vi "深大漂流记_main.vi"() -> ()   [LabVIEW 2018]
uses:
  <vilib>/Utility/file.llb/Read From Spreadsheet File (string).vi
panel:
  in  "富豪榜":i32[](listbox)
  out "leave":bool
  in  "关闭富豪榜":bool
  in  "查看富豪榜":bool
  in  "退出？":bool
  out "玩家":string caption="请输入你的大名"
  in  "放弃游戏":bool
  out "健康值":dbl(slide) scale=0.0..100.0
  out "当前健康值":i32=1000
  in  "医院":bool
  out "提示":string
  in  "信贷":bool
  out "欠债":i32
  in  "银行":bool
  out "存款":i32
  in  "演会中心":bool
  in  "机电学院":bool
  out "天数":i32
  out "余额":i32
  in  "饭堂":bool
  in  "图书馆":bool
  in  "库存":i32[](listbox)
  in  "卖出数量":i32 min=0 step=1
  in  "买入数量":i32 min=0 step=1
  in  "卖出":bool
  in  "买入":bool
  in  "商品价格":i32[](listbox)
  out "物品存在索引":i32[](array[numeric])
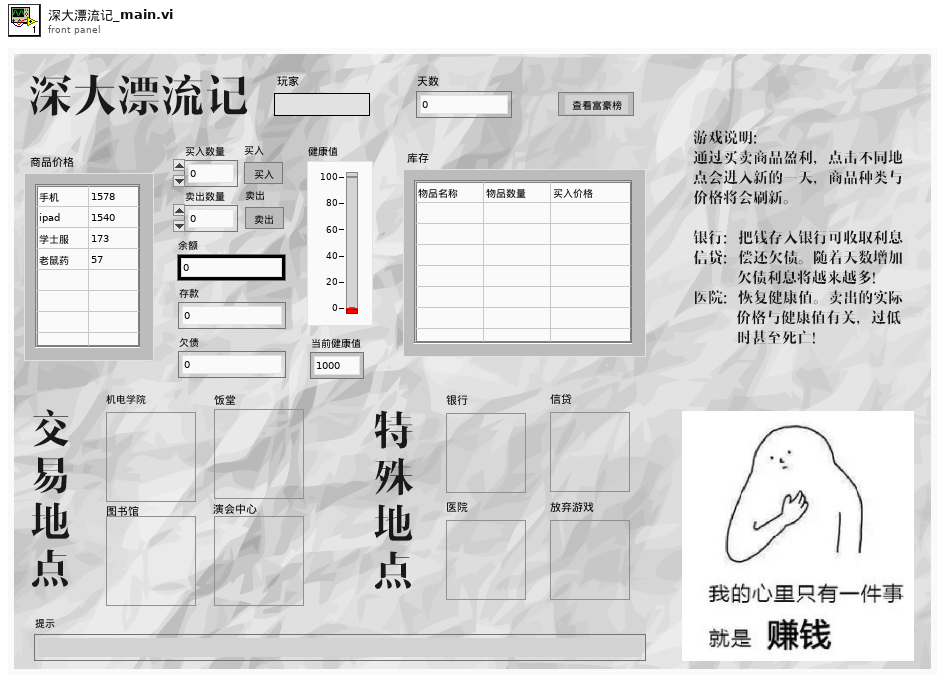
[diagram p1: front panel]
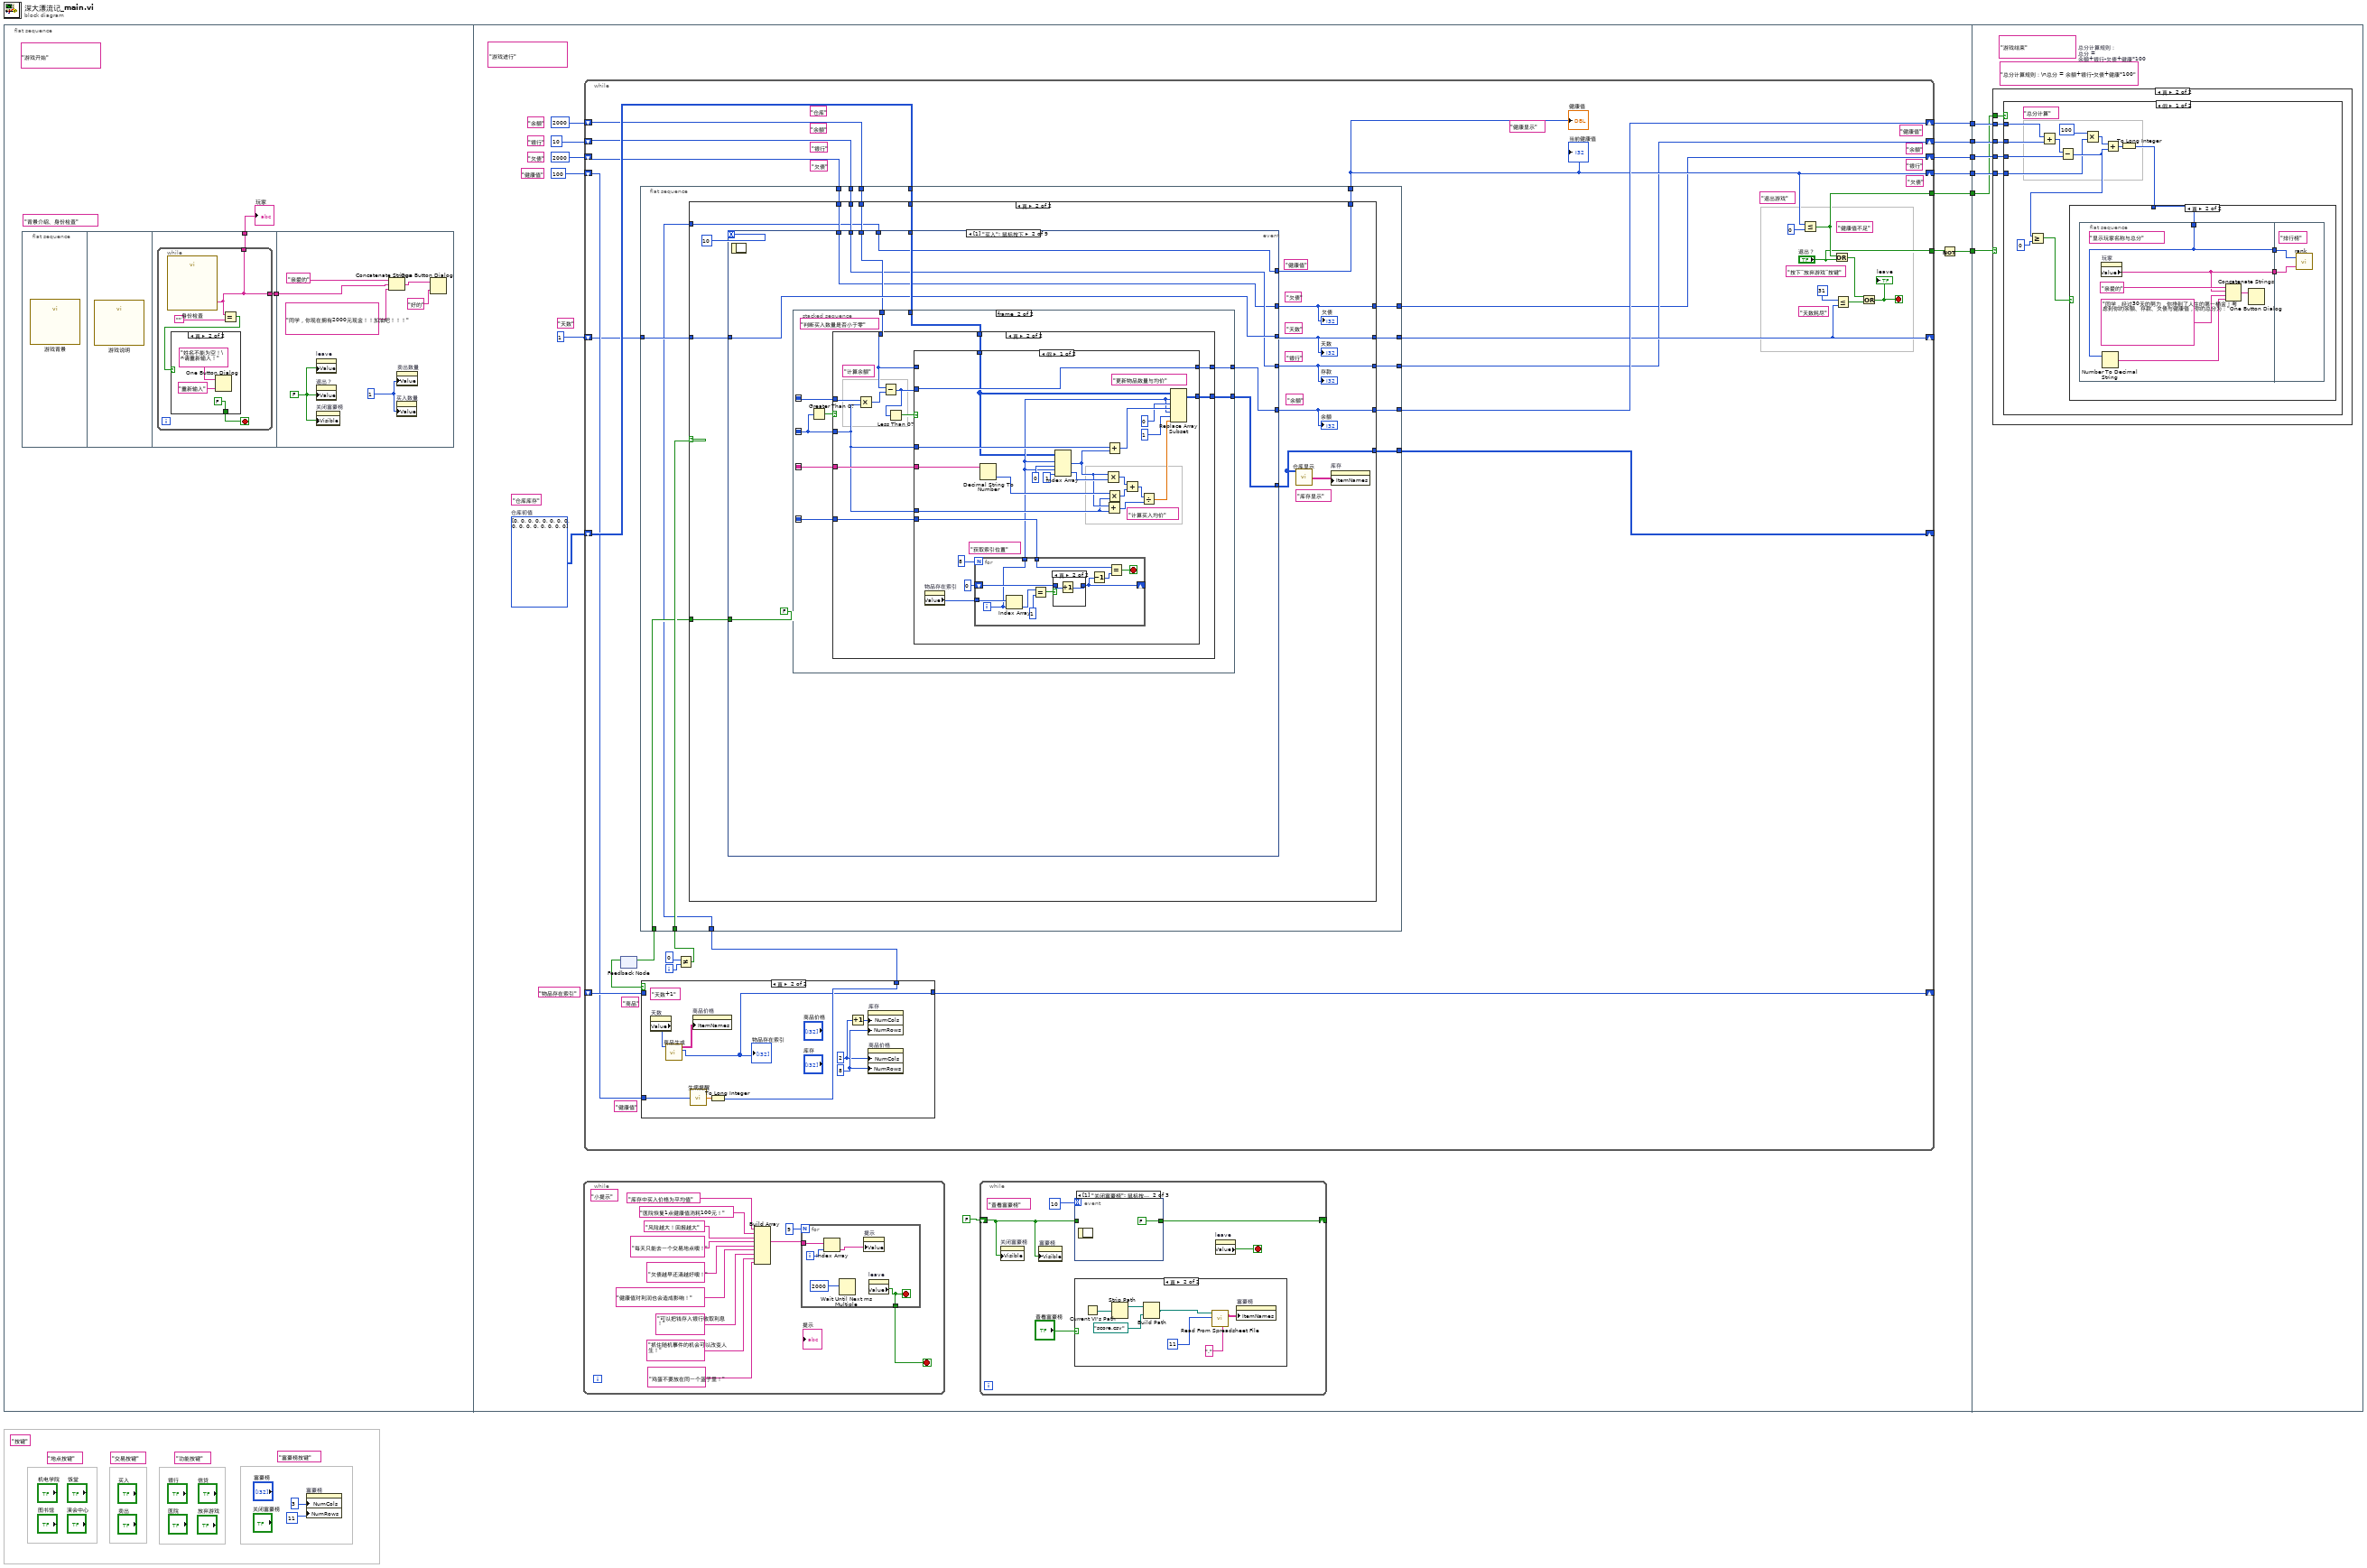
[diagram p0: block diagram]
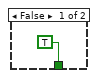
[diagram p2: hidden frame]
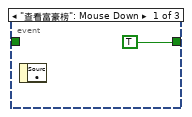
[diagram p3: hidden frame]
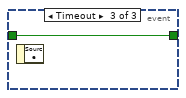
[diagram p4: hidden frame]
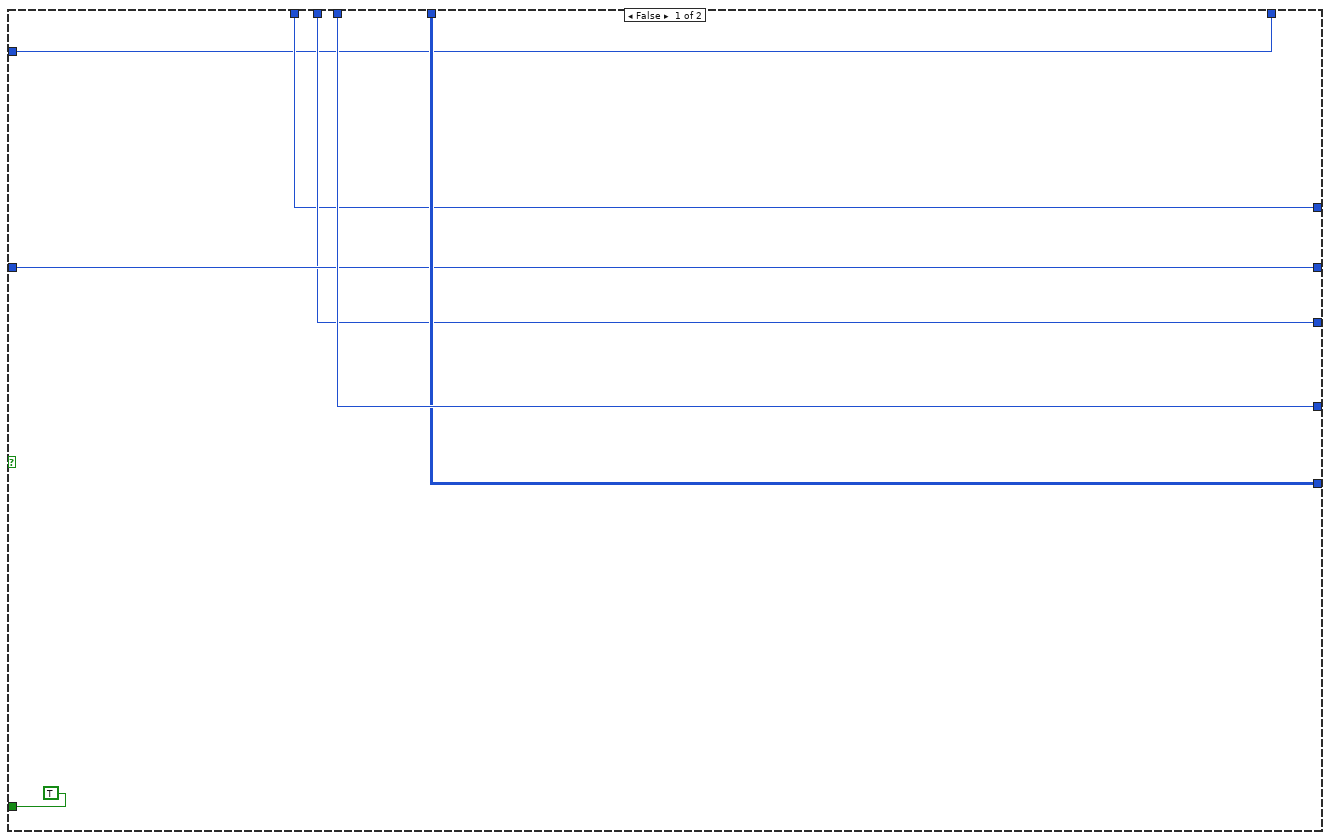
[diagram p7: hidden frame]
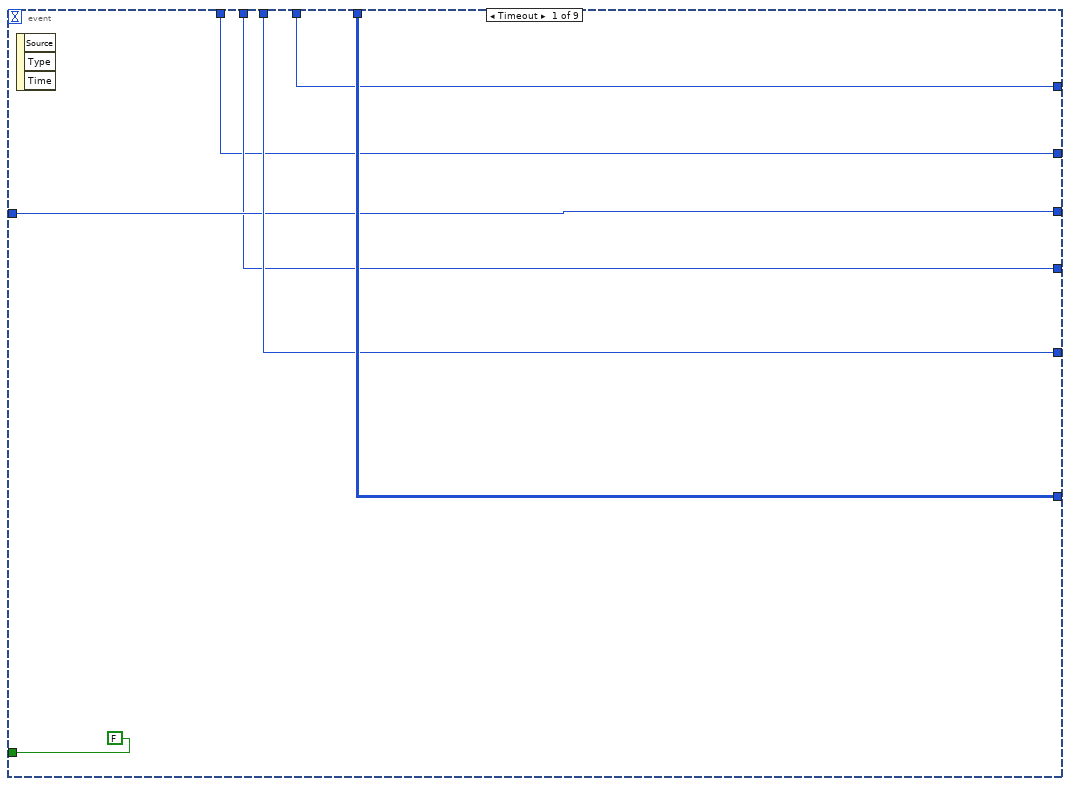
[diagram p8: hidden frame]
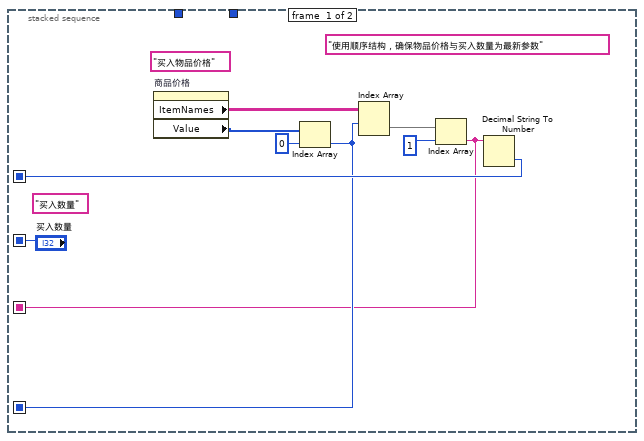
[diagram p9: hidden frame]
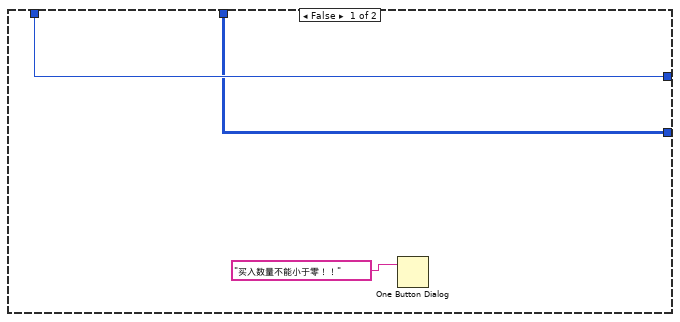
[diagram p10: hidden frame]
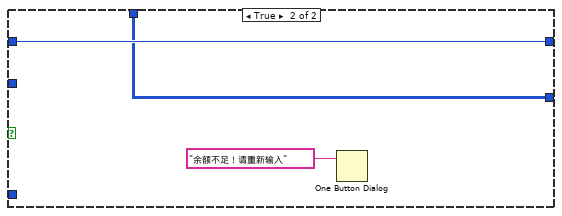
[diagram p12: hidden frame]
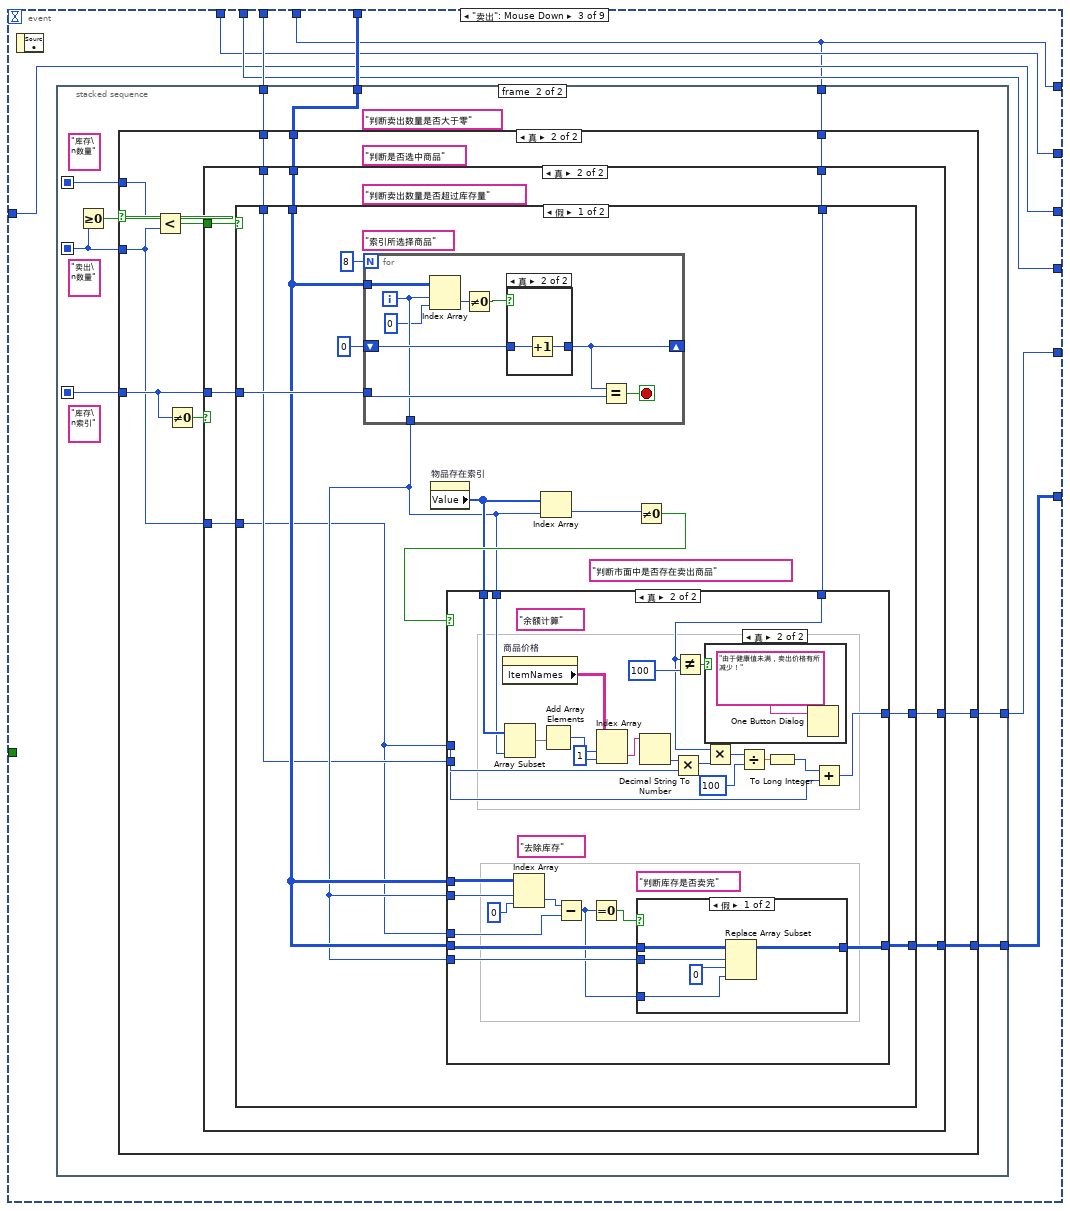
[diagram p13: hidden frame]
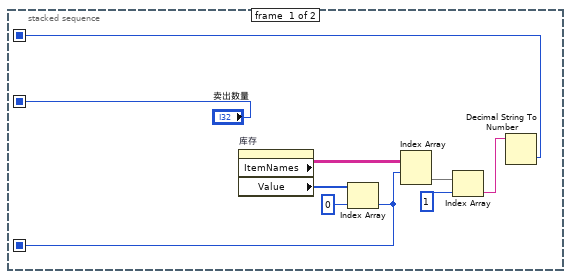
[diagram p14: hidden frame]
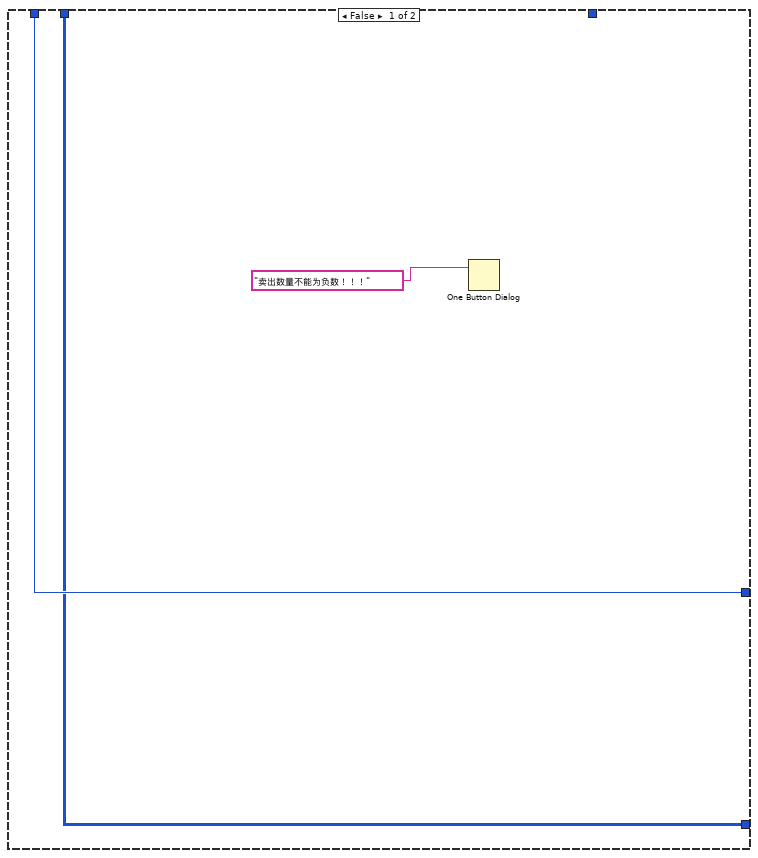
[diagram p15: hidden frame]
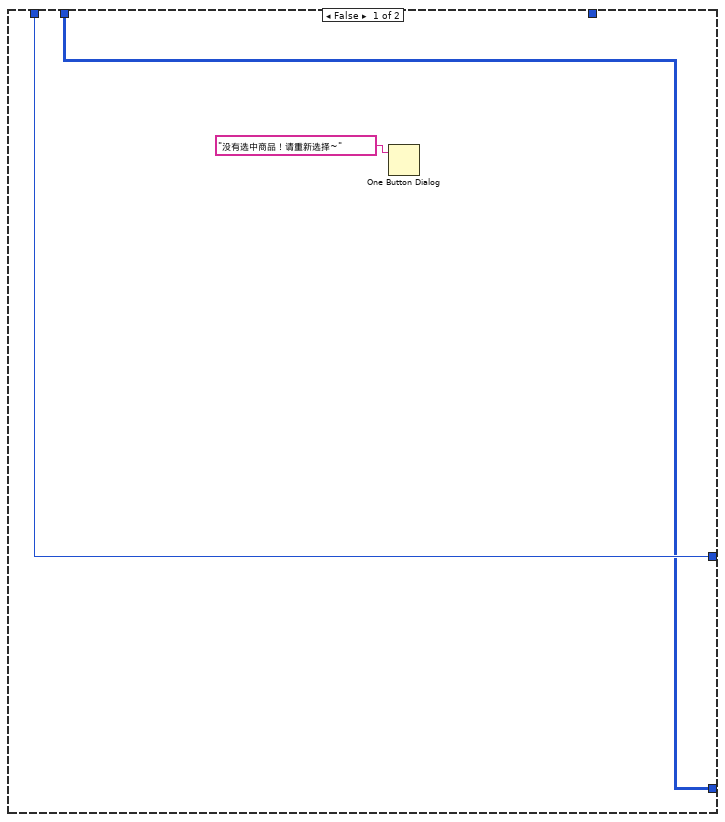
[diagram p16: hidden frame]
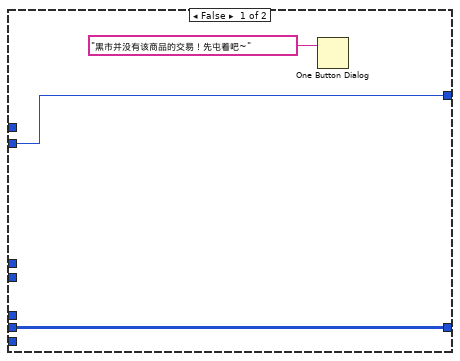
[diagram p17: hidden frame]
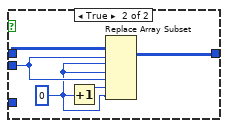
[diagram p19: hidden frame]
diagram:
  (unwired) "富豪榜按键"
  (unwired) "功能按键"
  (unwired) "交易按键"
  (unwired) "地点按键"
  (unwired) "按键"
  n1 = flat-sequence {
    tunnel: [w41] -> w8
    tunnel: [w40] -> w7
    tunnel: [w39] -> w6
    tunnel: [w38] -> w5
    tunnel: [w37] -> w4
    tunnel: [w28] -> w1
    tunnel: w8 -> [w522]
    tunnel: w7 -> [w521]
    tunnel: w6 -> [w520]
    tunnel: w5 -> [w519]
    tunnel: w4 -> [w518]
    tunnel: w1 -> [w517]
    frame #0 {
      (unwired) "背景介绍、身份检查"
      (unwired) "游戏开始"
      n2 = flat-sequence {
        tunnel: [w12] -> w10
        tunnel: [w11] -> w9
        tunnel: w10 -> [w26]
        frame #0 {
          n3 = call "游戏背景"() -> ()  [unwired: 18 in, 2 out]
        }
        frame #1 {
          n4 = call "游戏说明"() -> ()  [unwired: 18 in, 2 out]
        }
        frame #2 {
          n5 = while {
            tunnel: [w13] -> w12
            tunnel: [w13] -> w11
            stop <- w14 stop-if-true
            n6 = call "身份检查"() -> ("请输入你的姓名"=w13:string)  [unwired: 17 in, 2 out]
            n7 = Equal?(x=w13, y="") -> (x = y?=w15:bool)
            n8 = case shown="真" w15 {
              tunnel: [TRUE FALSE] -> w14
              frame False {
              }
              frame True {
                n9 = One Button Dialog(message="姓名不能为空！\n请重新输入！", button name ("OK")="重新输入" ("姓名输入提示")) -> ()  [unwired: 1 out]
              }
            }
          }
        }
        frame #3 {
          w21 = 1
          w22 = FALSE
          n10 = property on="leave" class="Bool (严格)"("Value"=w22) -> ()  [unwired: 2 in, 2 out]
          n11 = property on="退出？" class="Bool (严格)"("Value"=w22) -> ()  [unwired: 2 in, 2 out]
          n12 = property on="关闭富豪榜" class="Bool (严格)"("Visible"=w22) -> ()  [unwired: 2 in, 2 out]
          n13 = Concatenate Strings("亲爱的" ("姓名输入提示"), w26, "同学，你现在拥有2000元现金！！加油吧！！！" ("姓名输入提示")) -> (w24:string)
          n14 = property on="买入数量" class="DigNum (严格)"("Value"=w21) -> ()  [unwired: 2 in, 2 out]
          n15 = property on="卖出数量" class="DigNum (严格)"("Value"=w21) -> ()  [unwired: 2 in, 2 out]
          n16 = One Button Dialog(message=w24, button name ("OK")="好的" ("姓名输入提示")) -> ()  [unwired: 1 out]
        }
      }
      "玩家" <- w9
    }
    frame #1 {
      (unwired) "物品存在索引"
      (unwired) "游戏进行"
      (unwired) "健康值"
      (unwired) "欠债"
      (unwired) "银行"
      (unwired) "仓库库存"
      (unwired) "天数"
      (unwired) "余额"
      w32 = i32[][] [[0, 0], [0, 0], [0, 0], [0, 0], [0, 0], [0, 0], [0, 0], [0, 0]]  # 仓库初值
      n17 = while {
        stop <- w45 stop-if-true
        (unwired) "小提示"
        n18 = Build Array("库存中买入价格为平均值", "医院恢复1点健康值消耗100元！", "风险越大！回报越大", "每天只能去一个交易地点噢！", "欠债越早还清越好噢！", "健康值对利润也会造成影响！", "可以把钱存入银行收取利息！", "抓住随机事件的机会可以改变人生！", "鸡蛋不要放在同一个篮子里！") -> (w53:string[])
        n19 = for {
          N: 9 -> [_]
          tunnel: w53 -> [w58]
          tunnel: [w54] -> w45
          i -> [w57]
          stop <- w54 stop-if-true
          n20 = Index Array(array=w58, index=w57) -> (element=w55:string)
          n21 = Wait Until Next ms Multiple(millisecond multiple=2000) -> ()  [unwired: 1 out]
          n22 = property on="提示" class="Str"("Value"=w55) -> ()  [unwired: 2 in, 2 out]
          n23 = property on="leave" class="Bool (严格)"() -> ("Value"=w54:bool)  [unwired: 2 in, 2 out]
        }
      }
      n24 = while {
        shift-right: [w94] -> w41
        shift-left: 2000 -> [w87]
        shift-right: [w95] -> _
        shift-left: w32 -> [w96]
        shift-right: [w99] -> _
        shift-left: _ -> [w98]
        shift-right: [w91] -> _
        shift-left: 1 -> [w86]
        shift-right: [w79] -> w40
        shift-left: 10 -> [w88]
        shift-right: [w78] -> w39
        shift-left: 2000 -> [w89]
        shift-right: [w80] -> w38
        shift-left: 100 -> [w90]
        tunnel: [w81] -> w37
        tunnel: ["退出？"] -> w29
        i -> [w93]
        stop <- w84 stop-if-true
        (unwired) "天数耗尽"
        (unwired) "按下“放弃游戏”按键"
        (unwired) "健康值不足"
        (unwired) "退出游戏"
        (unwired) "健康显示"
        (unwired) "健康值"
        (unwired) "余额"
        (unwired) "银行"
        (unwired) "欠债"
        (unwired) "健康值"
        (unwired) "商品"
        (unwired) "仓库"
        (unwired) "余额"
        (unwired) "银行"
        (unwired) "欠债"
        n25 = feedback-in #1(w77) -> ()
        n26 = feedback #1() -> (w97:bool)  [unwired: 1 in]
        n27 = flat-sequence "平铺式顺序结构" {
          tunnel: w87 -> [w125]
          tunnel: [w121] -> w94
          tunnel: w76 -> [w124]
          tunnel: w96 -> [w123]
          tunnel: [w120] -> w95
          tunnel: [w122] -> w77
          tunnel: [w119] -> w91
          tunnel: w88 -> [w117]
          tunnel: [w116] -> w79
          tunnel: w89 -> [w115]
          tunnel: [w114] -> w78
          tunnel: [w113] -> w80
          tunnel: w75 -> [w112]
          tunnel: w86 -> [w118]
          frame #0 {
            n28 = case shown="真" w124 {
              tunnel: w125 -> [w132 w139]
              tunnel: [w132 w134] -> w121
              tunnel: w123 -> [w131 w146]
              tunnel: [w131 w144] -> w120
              tunnel: [TRUE w147] -> w122
              tunnel: [w129 w133] -> w119
              tunnel: w118 -> [w129 w142]
              tunnel: w117 -> [w128 w141]
              tunnel: [w128 w135] -> w116
              tunnel: w115 -> [w127 w140]
              tunnel: [w127 w136] -> w114
              tunnel: [w126 w138] -> w113
              tunnel: w112 -> [w126 w137]
              frame False {
              }
              frame True {
                (unwired) "库存显示"
                (unwired) "余额"
                (unwired) "天数"
                (unwired) "健康值"
                (unwired) "银行"
                (unwired) "欠债"
                n29 = event shown="[1] \"买入\": 鼠标按下" {
                  selector: _ -> [_ _ _ _ _ _ _ _ _]
                  dyn-events: _ -> [_ _ _ _ _ _ _ _ _]
                  timeout: 10 -> [_ _ _ _ _ _ _ _ _]
                  tunnel: [w152 w161 w242 w369 w378 w381 w447 w481 w512] -> w134
                  tunnel: w139 -> [w152 w158 w243 w369 w378 w386 w449 w482 w512]
                  tunnel: [w153 w162 w240 w370 w377 w382 w443 w486 w516] -> w144
                  tunnel: [FALSE FALSE _ TRUE FALSE _ _ _ _] -> w147
                  tunnel: w146 -> [w153 w163 w241 w370 w377 w382 w443 w486 w516]
                  tunnel: [w151 w159 w237 w365 w375 w380 w444 w483 w511] -> w133
                  tunnel: w142 -> [w151 w159 w237 w367 w375 w380 w444 w483 w511]
                  tunnel: w141 -> [w150 w157 w239 w357 w374 w385 w445 w484 w513]
                  tunnel: [w150 w157 w239 w358 w374 w384 w445 w484 w513] -> w135
                  tunnel: w140 -> [w149 w156 w238 w361 w373 w383 w448 w485 w514]
                  tunnel: [w149 w156 w238 w362 w373 w383 w446 w485 w514] -> w136
                  tunnel: w137 -> [w148 w155 w236 w366 w372 w379 w441 w478 w515]
                  tunnel: [w148 w155 w236 w366 w372 w379 w441 w477 w515] -> w138
                  event Timeout {
                    n30 = event-data() -> ()  [unwired: 1 in, 3 out]
                  }
                  event "买入": Mouse Down {
                    n31 = event-data() -> ()  [unwired: 1 in, 1 out]
                    n32 = stacked-sequence {
                      seq-local: ["买入数量" _] -> [_ w176]
                      seq-local: [w166 _] -> [_ w177]
                      seq-local: [w165 _] -> [_ w173]
                      seq-local: [w164 _] -> [_ w174]
                      tunnel: w158 -> [_ w181]
                      tunnel: w163 -> [_ w180]
                      tunnel: [_ w179] -> w162
                      tunnel: [_ w178] -> w161
                      frame #0 {
                        (unwired) "使用顺序结构，确保物品价格与买入数量为最新参数"
                        (unwired) "买入数量"
                        (unwired) "买入物品价格"
                        n33 = property on="商品价格" class="MCListbox (严格)"() -> ("ItemNames"=w169:string[][], "Value"=w168:i32[])  [unwired: 2 in, 2 out]
                        n34 = Index Array(array=w168, index=0) -> (element=w165:i32)
                        n35 = Index Array(array=w169, index (row)=w165) -> (element=w170:string[])  [unwired: 1 in]
                        n36 = Index Array(array=w170, index=1) -> (element=w164:string)
                        n37 = Decimal String To Number(string=w164) -> (number=w166:i32)  [unwired: 2 in, 1 out]
                      }
                      frame #1 {
                        (unwired) "判断买入数量是否小于零"
                        n38 = Greater Than 0?(x=w176) -> (x > 0?=w175:bool)
                        n39 = case shown="真" w175 {
                          tunnel: w181 -> [w183 w186]
                          tunnel: w174 -> [_ w194]
                          tunnel: w173 -> [_ w193]
                          tunnel: w180 -> [w182 w192]
                          tunnel: [w182 w191] -> w179
                          tunnel: [w183 w190] -> w178
                          tunnel: w177 -> [_ w189]
                          tunnel: w176 -> [_ w185]
                          frame False {
                            n40 = One Button Dialog(message="买入数量不能小于零！！") -> ()  [unwired: 1 in, 1 out]
                          }
                          frame True {
                            (unwired) "计算余额"
                            n41 = Multiply(x=w189, y=w185) -> (x*y=w195:i32)
                            n42 = Subtract(x=w186, y=w195) -> (x-y=w188:i32)
                            n43 = Less Than 0?(x=w188) -> (x < 0?=w187:bool)
                            n44 = case shown="假" w187 {
                              tunnel: [w219 w235] -> w190
                              tunnel: w188 -> [w219 _]
                              tunnel: w186 -> [_ w235]
                              tunnel: w194 -> [w213 _]
                              tunnel: w193 -> [w200 _]
                              tunnel: w192 -> [w196 w234]
                              tunnel: [w206 w234] -> w191
                              tunnel: w185 -> [w202 _]
                              tunnel: w185 -> [w199 _]
                              frame False {
                                (unwired) "更新物品数量与均价"
                                (unwired) "计算买入均价"
                                (unwired) "获取索引位置"
                                n45 = property on="物品存在索引" class="Arr (严格)"() -> ("Value"=w197:i32[])  [unwired: 2 in, 2 out]
                                n46 = for {
                                N: 8 -> [_]
                                tunnel: w197 -> [w229]
                                shift-right: [w225] -> _
                                shift-left: 0 -> [w226]
                                tunnel: w200 -> [w223]
                                tunnel: [w222] -> w198
                                i -> [w222]
                                stop <- w220 stop-if-true
                                n47 = Index Array(array=w229, index=w222) -> (element=w228:i32)
                                n48 = Equal?(x=w228, y=1) -> (x = y?=w221:bool)
                                n49 = case shown="真" w221 {
                                tunnel: w226 -> [w230 w232]
                                tunnel: [w230 w231] -> w225
                                frame False {
                                }
                                frame True {
                                n50 = Increment(x=w232) -> (x+1=w231:i32)
                                }
                                }
                                n51 = Decrement(x=w225) -> (x-1=w224:i32)
                                n52 = Equal?(x=w223, y=w224) -> (x = y?=w220:bool)
                                }
                                n53 = Decimal String To Number(string=w213) -> (number=w212:i32)  [unwired: 2 in, 1 out]
                                n54 = Index Array(array=w196, index (row) #1=w198, index (col) #1=0, index (row) #2=w198, index (col) #2=1) -> (element #1=w209:i32, element #2=w214:i32)
                                n55 = Multiply(x=w209, y=w214) -> (x*y=w211:i32)
                                n56 = Add(x=w209, y=w199) -> (x+y=w207:i32)
                                n57 = Add(x=w202, y=w209) -> (x+y=w216:i32)
                                n58 = Multiply(x=w212, y=w199) -> (x*y=w210:i32)
                                n59 = Add(x=w211, y=w210) -> (x+y=w208:i32)
                                n60 = Divide(x=w208, y=w207) -> (x/y=w203:dbl)
                                n61 = Replace Array Subset(array=w196, new element #1=w216, index (row) #1=w198, index (col) #1=0, new element #2=w203, index (row) #2=w198, index (col) #2=1) -> (w206:i32[][])
                              }
                              frame True {
                                n62 = One Button Dialog(message="余额不足！请重新输入") -> ()  [unwired: 1 in, 1 out]
                              }
                            }
                          }
                        }
                      }
                    }
                  }
                  event "卖出": Mouse Down {
                    n63 = event-data() -> ()  [unwired: 1 in, 1 out]
                    n64 = stacked-sequence {
                      seq-local: ["卖出数量" _] -> [_ w253]
                      seq-local: [w249 _] -> [_ w261]
                      seq-local: [w244 _] -> [_ w257]
                      tunnel: w241 -> [_ w260]
                      tunnel: w243 -> [_ w259]
                      tunnel: [_ w258] -> w242
                      tunnel: [_ w256] -> w240
                      tunnel: w236 -> [_ w255]
                      frame #0 {
                        n65 = property on="库存" class="MCListbox (严格)"() -> ("ItemNames"=w247:string[][], "Value"=w246:i32[])  [unwired: 2 in, 2 out]
                        n66 = Index Array(array=w246, index=0) -> (element=w244:i32)
                        n67 = Index Array(array=w247, index (row)=w244) -> (element=w248:string[])  [unwired: 1 in]
                        n68 = Index Array(array=w248, index=1) -> (element=w250:string)
                        n69 = Decimal String To Number(string=w250) -> (number=w249:i32)  [unwired: 2 in, 1 out]
                      }
                      frame #1 {
                        (unwired) "库存\n索引"
                        (unwired) "库存\n数量"
                        (unwired) "卖出\n数量"
                        (unwired) "判断卖出数量是否大于零"
                        n70 = Greater Or Equal To 0?(x=w253) -> (x >= 0?=w254:bool)
                        n71 = case shown="真" w254 {
                          tunnel: w261 -> [_ w274]
                          tunnel: w260 -> [w262 w272]
                          tunnel: w259 -> [w263 w271]
                          tunnel: [w263 w270] -> w258
                          tunnel: w257 -> [_ w269]
                          tunnel: w253 -> [_ w267]
                          tunnel: [w262 w266] -> w256
                          tunnel: w255 -> [_ w265]
                          frame False {
                            n72 = One Button Dialog(message="卖出数量不能为负数！！！") -> ()  [unwired: 1 in, 1 out]
                          }
                          frame True {
                            (unwired) "判断是否选中商品"
                            n73 = Less?(x=w274, y=w267) -> (x < y?=w273:bool)
                            n74 = Not Equal To 0?(x=w269) -> (x != 0?=w268:bool)
                            n75 = case shown="真" w268 {
                              tunnel: w273 -> [_ w281]
                              tunnel: w272 -> [w275 w285]
                              tunnel: w269 -> [_ w284]
                              tunnel: w267 -> [_ w283]
                              tunnel: w271 -> [w276 w278]
                              tunnel: [w276 w282] -> w270
                              tunnel: [w275 w280] -> w266
                              tunnel: w265 -> [_ w279]
                              frame False {
                                n76 = One Button Dialog(message="没有选中商品！请重新选择~") -> ()  [unwired: 1 in, 1 out]
                              }
                              frame True {
                                (unwired) "判断卖出数量是否超过库存量"
                                n77 = case shown="假" w281 {
                                tunnel: w285 -> [w291 w355]
                                tunnel: w284 -> [w296 _]
                                tunnel: w283 -> [w286 _]
                                tunnel: [w292 w354] -> w282
                                tunnel: [w289 w355] -> w280
                                tunnel: w279 -> [w288 _]
                                tunnel: w278 -> [w287 w354]
                                frame False {
                                (unwired) "判断市面中是否存在卖出商品"
                                (unwired) "索引所选择商品"
                                n78 = for {
                                N: 8 -> [_]
                                tunnel: w291 -> [w346]
                                shift-right: [w348] -> _
                                shift-left: 0 -> [w344]
                                tunnel: w296 -> [w345]
                                tunnel: [w343] -> w290
                                i -> [w343]
                                stop <- w347 stop-if-true
                                n79 = Index Array(array=w346, index (row)=w343, index (col)=0) -> (element=w350:i32)
                                n80 = Not Equal To 0?(x=w350) -> (x != 0?=w349:bool)
                                n81 = case shown="真" w349 {
                                tunnel: [w351 w353] -> w348
                                tunnel: w344 -> [w351 w352]
                                frame False {
                                }
                                frame True {
                                n82 = Increment(x=w352) -> (x+1=w353:i32)
                                }
                                }
                                n83 = Equal?(x=w348, y=w345) -> (x = y?=w347:bool)
                                }
                                n84 = property on="物品存在索引" class="Arr (严格)"() -> ("Value"=w293:i32[])  [unwired: 2 in, 2 out]
                                n85 = Index Array(array=w293, index=w290) -> (element=w295:i32)
                                n86 = Not Equal To 0?(x=w295) -> (x != 0?=w294:bool)
                                n87 = case shown="真" w294 {
                                tunnel: w290 -> [_ w329]
                                tunnel: w293 -> [_ w330]
                                tunnel: w286 -> [_ w324]
                                tunnel: w287 -> [w300 w323]
                                tunnel: [w300 w322] -> w292
                                tunnel: w291 -> [_ w320]
                                tunnel: w290 -> [_ w319]
                                tunnel: w286 -> [_ w317]
                                tunnel: w291 -> [w299 w314]
                                tunnel: w290 -> [_ w313]
                                tunnel: [w299 w312] -> w289
                                tunnel: w288 -> [_ w302]
                                frame False {
                                n88 = One Button Dialog(message="黑市并没有该商品的交易！先屯着吧~") -> ()  [unwired: 1 in, 1 out]
                                }
                                frame True {
                                (unwired) "判断库存是否卖完"
                                (unwired) "去除库存"
                                (unwired) "余额计算"
                                n89 = property on="商品价格" class="MCListbox (严格)"() -> ("ItemNames"=w327:string[][])  [unwired: 2 in, 2 out]
                                n90 = Array Subset(array=w330, length=w329) -> (w328:i32[])  [unwired: 1 in]
                                n91 = Index Array(array=w320, index (row)=w319, index (col)=0) -> (element=w316:i32)
                                n92 = Add Array Elements(numeric array=w328) -> (sum=w326:i32)
                                n93 = Subtract(x=w316, y=w317) -> (x-y=w311:i32)
                                n94 = Equal To 0?(x=w311) -> (x = 0?=w315:bool)
                                n95 = Index Array(array=w327, index (row)=w326, index (col)=1) -> (element=w307:string)
                                n96 = case shown="假" w315 {
                                tunnel: w314 -> [w336 w341]
                                tunnel: w313 -> [w335 w340]
                                tunnel: [w332 w337] -> w312
                                tunnel: w311 -> [w333 _]
                                frame False {
                                n97 = Replace Array Subset(array=w336, new element=w333, index (row)=w335, index (col)=0) -> (w332:i32[][])
                                }
                                frame True {
                                w338 = 0
                                n98 = Increment(x=w338) -> (x+1=w339:i32)
                                n99 = Replace Array Subset(array=w341, new element #1=w338, index (row) #1=w340, index (col) #1=w338, new element #2=w338, index (row) #2=w340, index (col) #2=w339) -> (w337:i32[][])
                                }
                                }
                                n100 = Decimal String To Number(string=w307) -> (number=w321:i32)  [unwired: 2 in, 1 out]
                                n101 = Multiply(x=w321, y=w324) -> (x*y=w310:i32)
                                n102 = Not Equal?(x=w302, y=100) -> (x != y?=w304:bool)
                                n103 = case shown="真" w304 {
                                frame False {
                                }
                                frame True {
                                n104 = One Button Dialog(message="由于健康值未满，卖出价格有所减少！") -> ()  [unwired: 1 in, 1 out]
                                }
                                }
                                n105 = Multiply(x=w302, y=w310) -> (x*y=w308:i32)
                                n106 = Divide(x=w308, y=100) -> (x/y=w306:dbl)
                                n107 = To Long Integer(number=w306) -> (32bit integer=w305:i32)
                                n108 = Add(x=w305, y=w323) -> (x+y=w322:i32)
                                }
                                }
                                }
                                frame True {
                                n109 = One Button Dialog(message="库存太少啦！请重新选择~") -> ()  [unwired: 1 in, 1 out]
                                }
                                }
                              }
                            }
                          }
                        }
                      }
                    }
                  }
                  event "图书馆", "机电学院", "演会中心", "饭堂": Mouse Up {
                    n110 = event-data() -> ()  [unwired: 1 in, 8 out]
                    n111 = Add(x=1, y=w367) -> (x+y=w365:i32)
                    n112 = Multiply(x=w357, y=1.05) -> (x*y=w359:dbl)
                    n113 = Multiply(x=w361, y=1.1) -> (x*y=w363:dbl)
                    n114 = To Long Integer(number=w359) -> (32bit integer=w358:i32)
                    n115 = To Long Integer(number=w363) -> (32bit integer=w362:i32)
                  }
                  event "库存", "商品价格": Mouse Down {
                    n116 = event-data() -> ()  [unwired: 1 in, 8 out]
                  }
                  event "银行": Mouse Down {
                    n117 = event-data() -> ()  [unwired: 1 in, 1 out]
                    n118 = Two Button Dialog(message="欢迎来到 IronBank ，你打算干什么？", 1:"取款", 2:"存款") -> (T button?=w387:bool)
                    n119 = case shown="假" w387 {
                      tunnel: w386 -> [w397 w421]
                      tunnel: w385 -> [w396 w420]
                      tunnel: [w395 w419] -> w381
                      tunnel: [w394 w418] -> w384
                      frame False {
                        (unwired) "取款"
                        n120 = call "输入取款数额"() -> ("取款数额"=w392:dbl)  [unwired: 17 in, 2 out]
                        n121 = To Long Integer(number=w392) -> (32bit integer=w391:i32)
                        n122 = Greater Or Equal To 0?(x=w391) -> (x >= 0?=w393:bool)
                        n123 = case shown="真" w393 {
                          tunnel: w397 -> [w400 w405]
                          tunnel: w396 -> [w399 w402]
                          tunnel: [w399 w404] -> w395
                          tunnel: [w400 w403] -> w394
                          tunnel: w391 -> [_ w401]
                          frame False {
                            n124 = One Button Dialog(message="取款数额必须大于等于0！") -> ()  [unwired: 1 in, 1 out]
                          }
                          frame True {
                            n125 = Less?(x=w402, y=w401) -> (x < y?=w406:bool)
                            n126 = case shown="假" w406 {
                              tunnel: [w411 w412] -> w404
                              tunnel: [w410 w413] -> w403
                              tunnel: w401 -> [w409 _]
                              tunnel: w405 -> [w408 w412]
                              tunnel: w402 -> [w407 w413]
                              frame False {
                                n127 = Subtract(x=w407, y=w409) -> (x-y=w410:i32)
                                n128 = Add(x=w408, y=w409) -> (x+y=w411:i32)
                              }
                              frame True {
                                n129 = One Button Dialog(message="余额不足！请重新输入") -> ()  [unwired: 1 in, 1 out]
                              }
                            }
                          }
                        }
                      }
                      frame True {
                        (unwired) "存款"
                        n130 = call "输入存款数额"() -> ("存款数额"=w416:dbl)  [unwired: 17 in, 2 out]
                        n131 = To Long Integer(number=w416) -> (32bit integer=w415:i32)
                        n132 = Greater Or Equal To 0?(x=w415) -> (x >= 0?=w417:bool)
                        n133 = case shown="真" w417 {
                          tunnel: w421 -> [w422 w429]
                          tunnel: w420 -> [w423 w428]
                          tunnel: [w422 w427] -> w419
                          tunnel: [w423 w426] -> w418
                          tunnel: w415 -> [_ w425]
                          frame False {
                            n134 = One Button Dialog(message="存款数额必须大于等于0！") -> ()  [unwired: 1 in, 1 out]
                          }
                          frame True {
                            n135 = Less?(x=w429, y=w425) -> (x < y?=w430:bool)
                            n136 = case shown="假" w430 {
                              tunnel: w425 -> [w435 _]
                              tunnel: [w434 w437] -> w427
                              tunnel: [w433 w436] -> w426
                              tunnel: w429 -> [w432 w437]
                              tunnel: w428 -> [w431 w436]
                              frame False {
                                n137 = Add(x=w431, y=w435) -> (x+y=w433:i32)
                                n138 = Subtract(x=w432, y=w435) -> (x-y=w434:i32)
                              }
                              frame True {
                                n139 = One Button Dialog(message="余额不足！请重新输入") -> ()  [unwired: 1 in, 1 out]
                              }
                            }
                          }
                        }
                      }
                    }
                  }
                  event "信贷": Mouse Down {
                    n140 = event-data() -> ()  [unwired: 1 in, 1 out]
                    n141 = call "输入还钱数额"() -> ("还钱数额"=w440:dbl)  [unwired: 17 in, 2 out]
                    n142 = To Long Integer(number=w440) -> (32bit integer=w439:i32)
                    n143 = Greater Or Equal To 0?(x=w439) -> (x >= 0?=w442:bool)
                    n144 = case shown="真" w442 {
                      tunnel: w449 -> [w451 w457]
                      tunnel: w439 -> [_ w456]
                      tunnel: w448 -> [w452 w455]
                      tunnel: [w451 w454] -> w447
                      tunnel: [w452 w453] -> w446
                      frame False {
                        n145 = One Button Dialog(message="输入必须大于等于0！") -> ()  [unwired: 1 in, 1 out]
                      }
                      frame True {
                        n146 = Less?(x=w457, y=w456) -> (x < y?=w458:bool)
                        n147 = case shown="假" w458 {
                          tunnel: w457 -> [w463 w475]
                          tunnel: w456 -> [w459 _]
                          tunnel: w455 -> [w462 w474]
                          tunnel: [w461 w475] -> w454
                          tunnel: [w460 w474] -> w453
                          frame False {
                            n148 = Less?(x=w462, y=w459) -> (x < y?=w464:bool)
                            n149 = case shown="假" w464 {
                              tunnel: w463 -> [w469 w473]
                              tunnel: w462 -> [w468 w472]
                              tunnel: [w466 w471] -> w461
                              tunnel: [w465 0] -> w460
                              tunnel: w459 -> [w467 _]
                              frame False {
                                n150 = Subtract(x=w469, y=w467) -> (x-y=w466:i32)
                                n151 = Subtract(x=w468, y=w467) -> (x-y=w465:i32)
                              }
                              frame True {
                                n152 = Subtract(x=w473, y=w472) -> (x-y=w471:i32)
                              }
                            }
                          }
                          frame True {
                            n153 = One Button Dialog(message="余额不足！请重新输入！") -> ()  [unwired: 1 in, 1 out]
                          }
                        }
                      }
                    }
                  }
                  event "医院": Mouse Down {
                    w479 = 100  # 健康初值
                    n154 = event-data() -> ()  [unwired: 1 in, 1 out]
                    n155 = Not Equal?(x=w479, y=w478) -> (x != y?=w480:bool)
                    n156 = case shown="真" w480 {
                      tunnel: w482 -> [w489 w494]
                      tunnel: [w489 w490] -> w481
                      tunnel: w478 -> [w487 w492]
                      tunnel: [w487 w491] -> w477
                      frame False {
                        n157 = One Button Dialog(message="没病来什么医院！" ("姓名输入提示")) -> ()  [unwired: 1 in, 1 out]
                      }
                      frame True {
                        w496 = 100  # 医院花费倍数
                        w498 = 100  # 健康初值
                        n158 = Subtract(x=w498, y=w492) -> (x-y=w497:i32)
                        n159 = Multiply(x=w497, y=w496) -> (x*y=w495:i32)
                        n160 = Greater Or Equal?(x=w494, y=w495) -> (x >= y?=w493:bool)
                        n161 = case shown="真" w493 {
                          tunnel: w494 -> [w500 w509]
                          tunnel: [w500 w508] -> w490
                          tunnel: w495 -> [_ w503]
                          tunnel: w492 -> [w499 _]
                          tunnel: [w499 100] -> w491
                          frame False {
                            n162 = One Button Dialog(message="没钱看什么病！" ("姓名输入提示")) -> ()  [unwired: 1 in, 1 out]
                          }
                          frame True {
                            n163 = Number To Decimal String(number=w503) -> (decimal integer string=w504:string)  [unwired: 1 in]
                            n164 = Subtract(x=w509, y=w503) -> (x-y=w508:i32)
                            n165 = Concatenate Strings("医生开了点药给您，共花费了" ("姓名输入提示"), w504, "元！" ("姓名输入提示")) -> (w507:string)
                            n166 = One Button Dialog(message=w507) -> ()  [unwired: 1 in, 1 out]
                          }
                        }
                      }
                    }
                  }
                  event "放弃游戏": Mouse Down {
                    n167 = event-data() -> ()  [unwired: 1 in, 1 out]
                    n168 = property on="退出？" class="Bool (严格)"("Value"=TRUE) -> ()  [unwired: 2 in, 2 out]
                  }
                }
                "余额" <- w134
                "天数" <- w133
                "存款" <- w135
                "欠债" <- w136
                n169 = call "仓库显示.vi"("仓库"=w144) -> ("显示栏"=w143:string[][])  [unwired: 10 in]
                n170 = property on="库存" class="MCListbox (严格)"("ItemNames"=w143) -> ()  [unwired: 2 in, 2 out]
              }
            }
          }
        }
        n171 = case shown="真" w97 {
          tunnel: [w102 w104] -> w99
          tunnel: w98 -> [w102 _]
          tunnel: w90 -> [w101 w108]
          tunnel: [w101 w106] -> w75
          frame False {
          }
          frame True {
            (unwired) "天数+1"
            w111 = i8 8
            w109 = i8 2
            n172 = property on="天数" class="DigNum (严格)"() -> ("Value"=w103:i32)  [unwired: 2 in, 2 out]
            n173 = call "商品生成.vi"("天数"=w103) -> ("物品存在索引"=w104:i32[], "市面商品"=w105:string[][])  [unwired: 9 in]
            "物品存在索引" <- w104
            n174 = call "生病提醒.vi"("数值"=w108) -> ("数值 2"=w107:dbl)
            n175 = property on="商品价格" class="MCListbox (严格)"("ItemNames"=w105) -> ()  [unwired: 2 in, 2 out]
            n176 = To Long Integer(number=w107) -> (32bit integer=w106:i32)
            n177 = Increment(x=w109) -> (x+1=w110:i8)
            n178 = property on="库存" class="MCListbox (严格)"("NumCols"=w110, "NumRows"=w111) -> ()  [unwired: 2 in, 2 out]
            n179 = property on="商品价格" class="MCListbox (严格)"("NumCols"=w109, "NumRows"=w111) -> ()  [unwired: 2 in, 2 out]
          }
        }
        n180 = Not Equal?(x=0, y=w93) -> (x != y?=w76:bool)
        n181 = Less Or Equal?(x=w80, y=0) -> (x <= y?=w81:bool)
        n182 = Or(x=w81, y="退出？") -> (x .or. y?=w82:bool)
        n183 = Less Or Equal?(x=31, y=w91) -> (x <= y?=w85:bool)
        n184 = Or(x=w82, y=w85) -> (x .or. y?=w84:bool)
        "leave" <- w84
        "当前健康值" <- w80
        "健康值" <- w80
      }
      n185 = while {
        shift-right: [w60] -> _
        shift-left: FALSE -> [w59]
        stop <- w61 stop-if-true
        (unwired) "查看富豪榜"
        n186 = property on="关闭富豪榜" class="Bool (严格)"("Visible"=w59) -> ()  [unwired: 2 in, 2 out]
        n187 = property on="富豪榜" class="MCListbox (严格)"("Visible"=w59) -> ()  [unwired: 2 in, 2 out]
        n188 = event shown="[1] \"关闭富豪榜\": 鼠标按下" {
          selector: _ -> [_ _ _]
          dyn-events: _ -> [_ _ _]
          timeout: 10 -> [_ _ _]
          tunnel: w59 -> [_ _ w66]
          tunnel: [TRUE FALSE w66] -> w60
          event "查看富豪榜": Mouse Down {
            n189 = event-data() -> ()  [unwired: 1 in, 1 out]
          }
          event "关闭富豪榜": Mouse Down {
            n190 = event-data() -> ()  [unwired: 1 in, 1 out]
          }
          event Timeout {
            n191 = event-data() -> ()  [unwired: 1 in, 1 out]
          }
        }
        n192 = case shown="真" "查看富豪榜" {
          frame False {
          }
          frame True {
            n193 = Current VI's Path() -> (path=w71:path)
            n194 = Strip Path(path=w71) -> (stripped path=w70:path)  [unwired: 1 out]
            n195 = Build Path(base path=w70, name or relative path=path "score.csv") -> (appended path=w68:path)
            n196 = call-poly <vilib>:"Read From Spreadsheet File.vi"("delimiter (\\t)"=",", "number of rows (all:-1)"=11, "file path (dialog if empty)"=w68) -> ("all rows"=w67:string[][])  [unwired: 4 in, 4 out]
            n197 = property on="富豪榜" class="MCListbox (严格)"("ItemNames"=w67) -> ()  [unwired: 2 in, 2 out]
          }
        }
        n198 = property on="leave" class="Bool (严格)"() -> ("Value"=w61:bool)  [unwired: 2 in, 2 out]
      }
      n199 = Not(x=w29) -> (.not. x?=w28:bool)
    }
    frame #2 {
      (unwired) "总分计算规则：\n总分 = 余额+银行-欠债+健康*100"  # 总分计算规则： 总分 = 余额+银行-欠债+健康*100
      (unwired) "游戏结束"
      n200 = case shown="真" w517 {
        tunnel: w522 -> [_ w531]
        tunnel: w521 -> [_ w530]
        tunnel: w520 -> [_ w529]
        tunnel: w519 -> [_ w528]
        tunnel: w518 -> [_ w527]
        frame False {
          n201 = property on="玩家" class="Str"() -> ("Value"=w523:string)  [unwired: 2 in, 2 out]
          n202 = Concatenate Strings("亲爱的", w523, "同学，你点击了放弃游戏！重新开始请点击”运行“按钮！") -> (w524:string)
          n203 = One Button Dialog(message=w524) -> ()  [unwired: 1 in, 1 out]
        }
        frame True {
          n204 = case shown="假" w527 {
            tunnel: w531 -> [w542 _]
            tunnel: w530 -> [w541 _]
            tunnel: w529 -> [w540 _]
            tunnel: w528 -> [w532 _]
            frame False {
              (unwired) "总分计算"
              n205 = Add(x=w542, y=w541) -> (x+y=w543:i32)
              n206 = Subtract(x=w543, y=w540) -> (x-y=w533:i32)
              n207 = Greater Or Equal?(x=w533, y=0) -> (x >= y?=w534:bool)
              n208 = Multiply(x=100, y=w532) -> (x*y=w537:i32)
              n209 = Add(x=w537, y=w533) -> (x+y=w539:i32)
              n210 = To Long Integer(number=w539) -> (32bit integer=w536:i32)
              n211 = case shown="真" w534 {
                tunnel: w536 -> [_ w548]
                frame False {
                  n212 = property on="玩家" class="Str"() -> ("Value"=w544:string)  [unwired: 2 in, 2 out]
                  n213 = Concatenate Strings("亲爱的", w544, "同学，你破产了！游戏结束！") -> (w545:string)
                  n214 = One Button Dialog(message=w545) -> ()  [unwired: 1 in, 1 out]
                }
                frame True {
                  n215 = flat-sequence {
                    tunnel: w548 -> [w551]
                    tunnel: [w552] -> w550
                    tunnel: [w551] -> w549
                    tunnel: w550 -> [w558]
                    tunnel: w549 -> [w557]
                    frame #0 {
                      (unwired) "显示玩家名称与总分"
                      n216 = property on="玩家" class="Str"() -> ("Value"=w552:string)  [unwired: 2 in, 2 out]
                      n217 = Number To Decimal String(number=w551) -> (decimal integer string=w554:string)  [unwired: 1 in]
                      n218 = Concatenate Strings("亲爱的", w552, "同学，经过30天的努力，你挣到了人生的第一桶金！考虑到你的余额、存款、欠债与健康值，你的总分为：", w554) -> (w553:string)
                      n219 = One Button Dialog(message=w553) -> ()  [unwired: 1 in, 1 out]
                    }
                    frame #1 {
                      (unwired) "排行榜"
                      n220 = call "rank.vi"("玩家名称"=w558, "得分"=w557) -> ()  [unwired: 1 in]
                    }
                  }
                }
              }
            }
            frame True {
              n221 = property on="玩家" class="Str"() -> ("Value"=w559:string)  [unwired: 2 in, 2 out]
              n222 = Concatenate Strings("亲爱的", w559, "同学，你的健康值低于0，游戏结束！") -> (w560:string)
              n223 = One Button Dialog(message=w560) -> ()  [unwired: 1 in, 1 out]
            }
          }
        }
      }
    }
  }
  n224 = property on="富豪榜" class="MCListbox (严格)"("NumCols"=3, "NumRows"=11) -> ()  [unwired: 2 in, 2 out]
